vi "to_json.vi"(8 "error in":errorcluster, 11 "ts.epochOfTimeUnit in":refnum<class "ts.epochOfTimeUnit.lvclass">) -> (0 "error out":errorcluster, 2 "json":string, 3 "ts.epochOfTimeUnit out":refnum<class "ts.epochOfTimeUnit.lvclass">, 4 "Not Default":bool)   [LabVIEW 2020, in "ts.epochOfTimeUnit.lvclass"]
uses:
  ts.epochOfTimeUnit.lvclass
  ts.epochOfTimeUnit.lvclass/ts.epochOfTimeUnit.ctl
  ed7ab10c-43ce-4bfb-94be-fb360c416495.vi
  8228e4ca-03be-40b8-987d-2b8b2c52d251.vi
  2851d703-dd12-49b4-904f-bee0f4943dab.vi
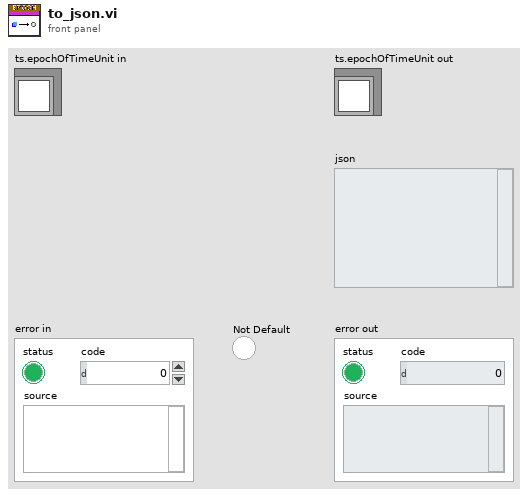
[diagram p1: front panel]
types:
  T1 = enum16{"DAYS", "HOURS", "MINUTES", "SECONDS", "MILLISECONDS", "MICROSECONDS", "NANOSECONDS", "PICOSECONDS"}
  T2 = cluster{"type":string, "epochOfTimeUnit":cluster{"timeUnit":string}}
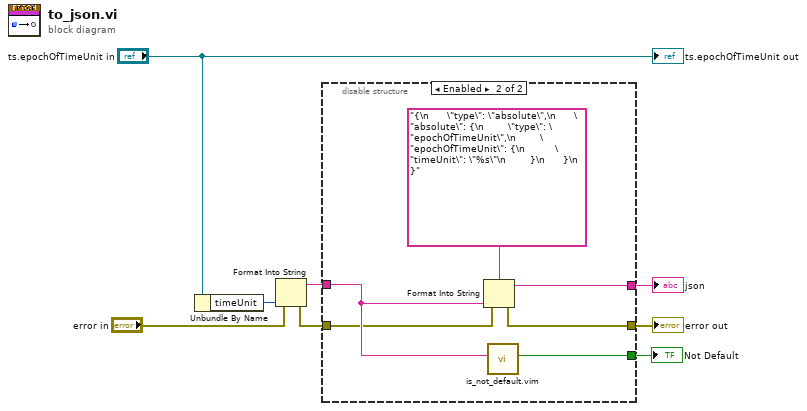
[diagram p0: block diagram]
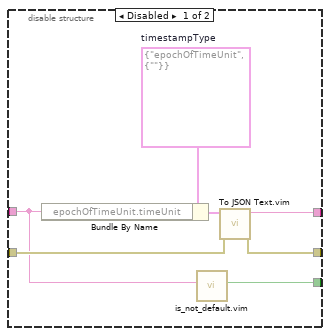
[diagram p2: hidden frame]
diagram:
  n1 = Unbundle By Name("ts.epochOfTimeUnit in") -> ("timeUnit"=w8:T1)
  n2 = Format Into String(error in="error in", w8) -> (resulting string=w2:string, error out=w6:errorcluster)  [unwired: 2 in]
  n3 = disable-structure shown="Enabled" {
    disable-tunnel: w6 -> [w13 w18]
    disable-tunnel: [w12 w19] -> w5
    disable-tunnel: [w11 w17] -> w4
    disable-tunnel: w2 -> [w10 w20]
    disable-tunnel: [w9 w16] -> w1
    frame Disabled {
      w15 = T2 {"type"="epochOfTimeUnit", "epochOfTimeUnit"={"timeUnit"=""}}  # timestampType
      n4 = Bundle By Name(cluster=w15, "epochOfTimeUnit.timeUnit"=w10) -> (w14:T2)
      n5 = call "is_not_default.vim"("data"=w10) -> ("Not Default"=w9:bool)  [unwired: 10 in]
      n6 = call "To JSON Text.vim"("error in (no error)"=w13, "Anything"=w14) -> ("error out"=w12:errorcluster, "<JSON>"=w11:string)  [unwired: 8 in]
    }
    frame Enabled {
      n7 = Format Into String(format string="{\n      \"type\": \"absolute\",\n      \"absolute\": {\n        \"type\": \"epochOfTimeUnit\",\n        \"epochOfTimeUnit\": {\n          \"timeUnit\": \"%s\"\n        }\n      }\n    }", error in=w18, w20) -> (resulting string=w17:string, error out=w19:errorcluster)  [unwired: 1 in]
      n8 = call "is_not_default.vim"("data"=w20) -> ("Not Default"=w16:bool)  [unwired: 10 in]
    }
  }
  "error out" <- w5
  "json" <- w4
  "Not Default" <- w1
  "ts.epochOfTimeUnit out" <- "ts.epochOfTimeUnit in"
